vi "Get Slew Rates.vi"(6 "error in (no error)":errorcluster {"code" format="%.0x"}, 9 "instrument handle":refnum<visa-resource-name>) -> (0 "error out":errorcluster {"code" format="%.0x"}, 1 "power slew rate":sgl, 2 "current slew rate":sgl, 3 "instrument handle out":refnum<visa-resource-name>, 4 "resistance slew rate":sgl, 5 "voltage slew rate":sgl)   [LabVIEW 2018]
uses:
  <instrlib>/NHRDCPowerModule/NHRDCPowerModule/NHRDCPowerModule.lvlib
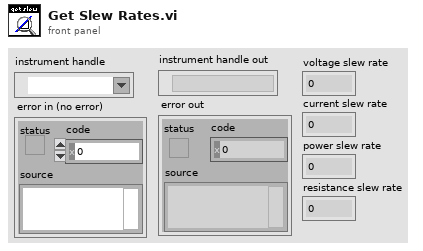
[diagram p1: front panel]
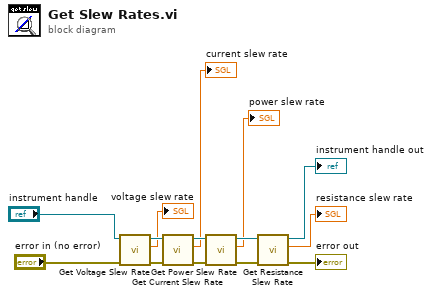
[diagram p0: block diagram]
diagram:
  n1 = call <instrlib>:"Get Voltage Slew Rate.vi"("error in (no error)"="error in (no error)", "instrument handle"="instrument handle") -> ("error out"=w11:errorcluster, "voltage slew rate"=→"voltage slew rate":sgl, "instrument handle out"=w14:refnum<visa-resource-name>)  [unwired: 7 in]
  n2 = call <instrlib>:"Get Current Slew Rate.vi"("error in (no error)"=w11, "instrument handle"=w14) -> ("error out"=w10:errorcluster, "current slew rate"=→"current slew rate":sgl, "instrument handle out"=w13:refnum<visa-resource-name>)  [unwired: 7 in]
  n3 = call <instrlib>:"Get Power Slew Rate.vi"("error in (no error)"=w10, "instrument handle"=w13) -> ("error out"=w9:errorcluster, "power slew rate"=→"power slew rate":sgl, "instrument handle out"=w12:refnum<visa-resource-name>)  [unwired: 7 in]
  n4 = call <instrlib>:"Get Resistance Slew Rate.vi"("error in (no error)"=w9, "instrument handle"=w12) -> ("error out"=→"error out":errorcluster, "resistance slew rate"=→"resistance slew rate":sgl, "instrument handle out"=→"instrument handle out":refnum<visa-resource-name>)  [unwired: 7 in]
